vi "test-ppms-test-factory.vi"() -> ()   [LabVIEW 2019]
uses:
  <userlib>/LevyLab/Instrument Framework/Instrument UI/Instrument UI.lvclass
  lvsrc/instrument.PPMS UI/Instrument UI.PPMS.lvclass
  lvsrc/PPMS/PPMS.lvlib
  <vilib>/JKI/JKI SMO/SMO/SMO.lvclass
  <vilib>/addons/_JKI Toolkits/Caraya/classes/Test/Test.lvclass
  <vilib>/addons/_JKI Toolkits/Caraya/classes/Assert/Assert.lvclass
  <vilib>/addons/_JKI Toolkits/Caraya/classes/Assert/Assert Equal Value_Variant.vi
  C:/Program Files (x86)/National Instruments/LabVIEW 2019/user.lib/LevyLab/Instrument Framework/Instrument UI/Instrument UI.lvclass
  C:/Program Files (x86)/National Instruments/LabVIEW 2019/vi.lib/JKI/JKI SMO/SMO/SMO.lvclass
  lvsrc/PPMS/Select PPMS--Enum.ctl
  lvsrc/instrument.PPMS/instrument.PPMS.lvclass
  C:/Program Files (x86)/National Instruments/LabVIEW 2019/user.lib/LevyLab/Instrument Framework/Instrument/Instrument.lvclass
panel:
  out "Select PPMS out":T1
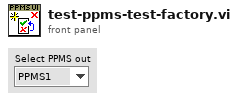
[diagram p1: front panel]
types:
  T1 = typedef "PPMS.lvlib/Select PPMS--Enum.ctl" = enum16{"PPMS1", "PPMS2", "PPMS3", "OptiCool", "Simulate PPMS", "Simulate OptiCool"}
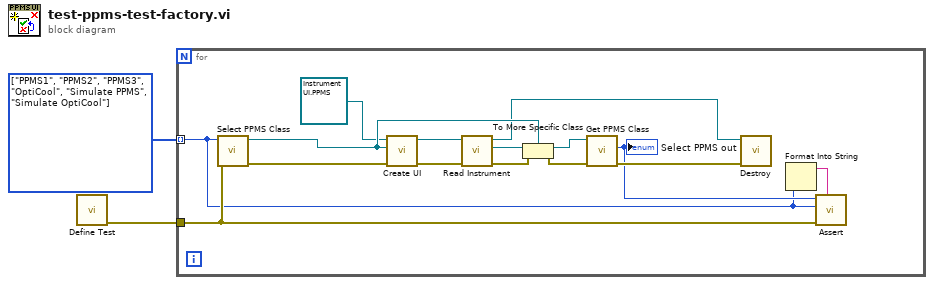
[diagram p0: block diagram]
diagram:
  w2 = T1[] [enum."PPMS1", enum."PPMS2", enum."PPMS3", enum."OptiCool", enum."Simulate PPMS", enum."Simulate OptiCool"] items=["PPMS1", "PPMS2", "PPMS3", "OptiCool", "Simulate PPMS", "Simulate OptiCool"] ("Array")
  n1 = call <vilib>:"Define Test.vi"() -> ("error out"=w1:errorcluster)  [unwired: 10 in, 1 out]
  n2 = for {
    tunnel: w2 -> [w4] mode=indexing
    tunnel: w1 -> [w5]
    n3 = call "Select PPMS Class.vi"("error in (no error)"=w5, "Select PPMS"=w4) -> ("error out"=w17:errorcluster, "instrument.PPMS out"=w16:refnum<class "instrument.PPMS.lvclass">)  [unwired: 8 in]
    n4 = call <userlib>:"Create UI.vi"("error in (no error)"=w17, "Instrument in"=w16, "Instrument UI"=refnum<class "Instrument UI.PPMS.lvclass"> refnum ("SR7220 UI.lvclass")) -> ("error out"=w8:errorcluster, "Instrument UI out"=w9:refnum<class "Instrument UI.PPMS.lvclass">)  [unwired: 7 in]
    n5 = call <userlib>:"Read Instrument.vi"("error in (no error)"=w8, "Instrument UI in"=w9) -> ("error out"=w7:errorcluster, "Instrument"=w6:refnum<class "Instrument.lvclass">, "Instrument UI"=w12:refnum<class "Instrument UI.PPMS.lvclass">)  [unwired: 7 in]
    n6 = To More Specific Class(target class=w16, reference=w6, error in=w7) -> (specific class reference=w15:refnum<class "instrument.PPMS.lvclass">, error out=w14:errorcluster)
    n7 = call "Get PPMS Class.vi"("error in (no error)"=w14, "instrument.PPMS"=w15) -> ("error out"=w13:errorcluster, "Select PPMS"=w11:T1)  [unwired: 7 in, 1 out]
    "Select PPMS out" <- w11
    n8 = call <vilib>:"Destroy.vi"("error in (no error)"=w13, "SMO"=w12) -> ()  [unwired: 9 in, 1 out]
    n9 = Format Into String(w4) -> (resulting string=w3:string)  [unwired: 3 in, 1 out]
    n10 = call-poly <vilib>:"Assert.vi"("Label"=w3, "error in (no error)"=w5, "Actual"=w4, "Expected"=w11) -> ()  [unwired: 6 in, 2 out]
  }
